vi "TestObservePath_ValueCFolderFileDotExt.vi"(8 "error in (no error)":errorcluster, 11 "TestCase in":refnum<class "TestObservableData.lvclass">) -> (0 "error out":errorcluster, 3 "TestCase out":refnum<class "TestObservableData.lvclass">)   [LabVIEW 2015, in "TestObservableData.lvclass"]
uses:
  TestObservableData.lvclass
  TestObservableData.lvclass/TestObservableData.ctl
  Framework/IMediator/IMediator Messages/Subscribe Msg/Subscribe Msg.lvclass/Subscribe Msg.ctl
  <vilib>/ActorFramework/Message Enqueuer/Message Enqueuer.lvclass/Message Enqueuer.ctl
  <vilib>/ActorFramework/Message Enqueuer/Enqueue.vi
  <vilib>/ActorFramework/Message Priority Queue/Priority Enqueue.vi
  Framework/IMediator/IMediator Messages/Subscribe Msg/Subscribe Msg.lvclass
  Framework/IMediator/SubscriptionRequest/SubscriptionRequest.lvclass
  Framework/IMediator/ISubscriptionPolicy/ISubscriptionPolicy.lvclass
  Framework/Mediator/Transport/TerminalBinding/TerminalBinding.lvclass
panel:
  out "ControlTerminal":path
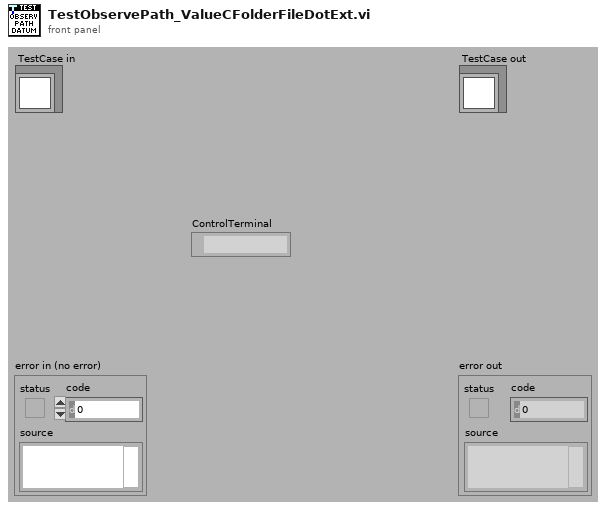
[diagram p1: front panel]
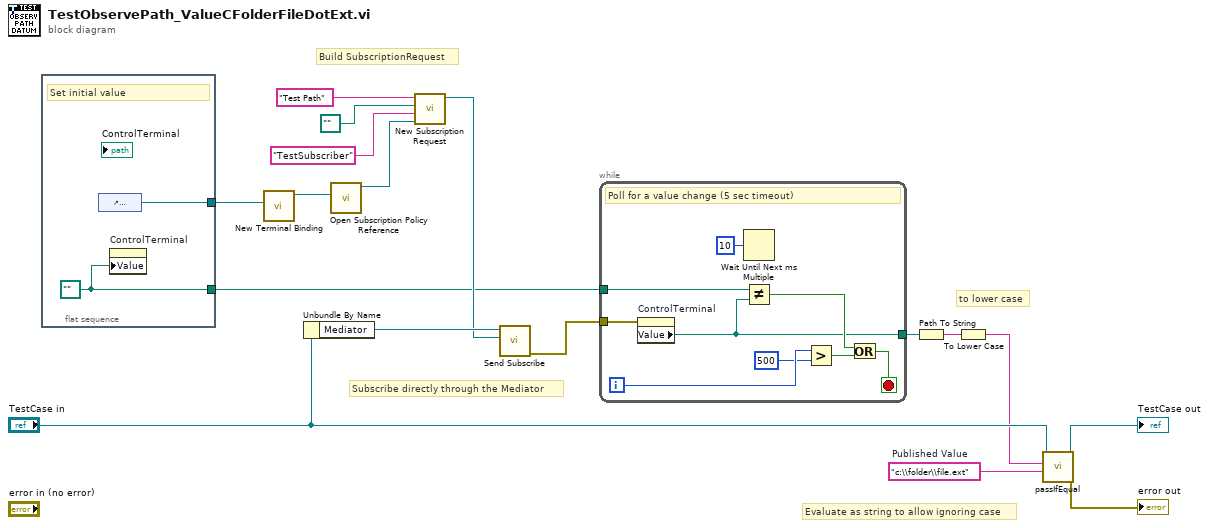
[diagram p0: block diagram]
diagram:
  w3 = "c:\\folder\\file.ext"  # Published Value
  # "to lower case"
  # "Evaluate as string to allow ignoring case"
  # "Build SubscriptionRequest"
  # "Subscribe directly through the Mediator"
  n1 = flat-sequence {
    tunnel: [w19] -> w7
    tunnel: [w18] -> w5
    frame #0 {
      w18 = path "" ("ControlTerminal")
      # "Set initial value"
      n2 = control-ref of="ControlTerminal"() -> (w19:refnum<vi>)
      n3 = property on="ControlTerminal" class="Path"("Value"=w18) -> ()  [unwired: 2 in, 2 out]
    }
  }
  n4 = call "New Terminal Binding.vi"("Ctl Refnum"=w7) -> ("TerminalBinding out"=w8:refnum<class "TerminalBinding.lvclass">)  [unwired: 9 in, 1 out]
  n5 = Unbundle By Name("TestCase in") -> ("Mediator"=w14:refnum<class "Message Enqueuer.lvclass">)
  n6 = call "Open Subscription Policy Reference.vi"("Transport"=w8) -> ("Subscription Policy"=w9:refnum<data-value>)  [unwired: 9 in, 1 out]
  n7 = call "New Subscription Request.vi"("Subscription Policy"=w9, "Unique Subscriber ID"="TestSubscriber", "Type"=path "", "Topic Name"="Test Path") -> ("SubscriptionRequest"=w13:refnum<class "SubscriptionRequest.lvclass">)  [unwired: 7 in]
  n8 = call "Send Subscribe.vi"("Subscription Request"=w13, "Message Enqueuer"=w14) -> ("error out"=w6:errorcluster)  [unwired: 8 in, 1 out]
  n9 = while {
    tunnel: w6 -> [w28]
    tunnel: w5 -> [w27]
    tunnel: [w20] -> w4
    i -> [w23]
    stop <- w21 stop-if-true
    # "Poll for a value change (5 sec timeout)"
    n10 = property on="ControlTerminal" class="Path"(error in=w28) -> ("Value"=w20:path)  [unwired: 1 in, 2 out]
    n11 = Wait Until Next ms Multiple(millisecond multiple=u32 10 ("milliseconds to wait")) -> ()  [unwired: 1 out]
    n12 = Not Equal?(x=w27, y=w20) -> (x != y?=w26:bool)
    n13 = Greater?(x=w23, y=500) -> (0:w24:bool)
    n14 = Or(x=w26, y=w24) -> (x .or. y?=w21:bool)
  }
  n15 = Path To String(path=w4) -> (string=w2:string)
  n16 = To Lower Case(string=w2) -> (all lower case string=w1:string)
  n17 = call-dynamic "passIfEqual.vi"("y"=w3, "x"=w1, "TestCase in"="TestCase in") -> ("error out"=→"error out":errorcluster, "TestCase out"=→"TestCase out":refnum<class "TestObservableData.lvclass">)  [unwired: 7 in]
